vi "Teleop.vi"(10 "Match Info":T1={"Autonomous Elapsed Seconds"=0.0, "TeleOp Elapsed Seconds"=0.0, "Disabled Elapsed Seconds"=0.0, "Visited Autonomous"=FALSE, "Visited TeleOp"=FALSE, "Visited Disabled"=FALSE, "Autonomous Settings"={"Autonomous Style"=enum."Independent", "VI Refnum"=refnum}}, 11 "Call Context":T2) -> ()   [LabVIEW 2017]
doc: "This VI is called for each TeleOp packet received from the DS where the robot is not disabled. It is often used to read from the joysticks and update I/O or to update setpoints for timed control loops. It should complete and return within 20 milliseconds or it may miss DS packets."
uses:
  <vilib>/Rock Robotics/WPI/DriverStation/WPI_DriverStationDerivedRobotMode.ctl
  <vilib>/Rock Robotics/WPI/DriverStation/WPI_DriverStationMatch Info.ctl
  globals.vi
  <vilib>/Rock Robotics/WPI/Utilities/WPI_GetSetVariantRefNum.vi
  <vilib>/Rock Robotics/Network Tables/NT Write Boolean Array.vi
  <vilib>/Rock Robotics/Network Tables/NT Write Numeric Array.vi
  <vilib>/Rock Robotics/Network Tables/NT Read Boolean.vi
  <vilib>/Rock Robotics/Network Tables/NT Read Number.vi
panel:
  out "Sample Slider 0":dbl(slide) scale=0.0..5.0
  out "Sample Boolean 1":bool
  out "Sample Boolean 0":bool
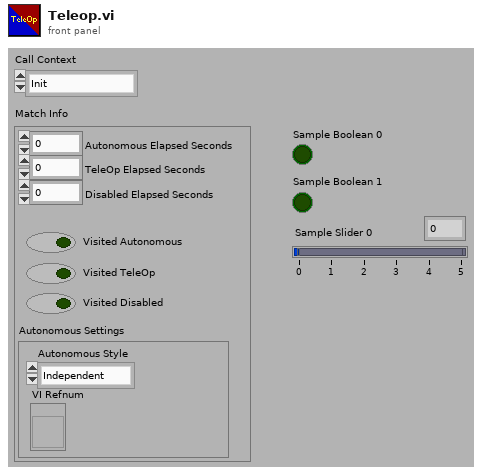
[diagram p1: front panel]
types:
  T1 = typedef "WPI_DriverStationMatch Info.ctl" = cluster{"Autonomous Elapsed Seconds":dbl, "TeleOp Elapsed Seconds":dbl, "Disabled Elapsed Seconds":dbl, "Visited Autonomous":bool, "Visited TeleOp":bool, "Visited Disabled":bool, "Autonomous Settings":cluster{"Autonomous Style":enum16{"Iterative", "Independent"}, "VI Refnum":refnum<vi>}}
  T2 = typedef "WPI_DriverStationDerivedRobotMode.ctl" = enum16{"Init", "Execute", "Stop"}
  T3 = typedef "WPI_JoystickDevRef.ctl" = cluster{"Device":T4}
  T4 = typedef "WPI_JoystickDeviceEnum.ctl" = enum16{"USB 0", "USB 1", "USB 2", "USB 3", "USB 4", "USB 5"}
  T5 = typedef "WPI_MotorControlDeviceRef.ctl" = cluster{"DeviceStatus":errorcluster, "Type":T6, "PWM":cluster{"PWM Channel":T7, "DeadBand":T8}, "CAN":cluster{"Device Number":u8, "SetOutput VI Ref":variant, "GetOutput VI Ref":variant, "Enable VI Ref":variant, "Disable VI Ref":variant, "Data":variant}, "Invert":bool, "DIO PWM":cluster{"PWM \"Enable\" Channel":T7, "DIOChannel":T9, "PWM Rate":dbl}}
  T6 = typedef "WPI_MotorControlType.ctl" = enum16{"PWM", "CAN", "DIO PWM"}
  T7 = typedef "FPGA_DIOPWMChannel.ctl" = enum8{"PWM 0", "PWM 1", "PWM 2", "PWM 3", "PWM 4", "PWM 5", "PWM 6", "PWM 7", "PWM 8", "PWM 9", "PWM MXP 0", "PWM MXP 1", "PWM MXP 2", "PWM MXP 3", "PWM MXP 4", "PWM MXP 5", "PWM MXP 6", "PWM MXP 7", "PWM MXP 8", "PWM MXP 9", "Invalid"}
  T8 = typedef "WPI_PWMDeadband.ctl" = cluster{"Name":string, "maxPositivePwm":i32, "minPositivePwm":i32, "centerPwm":i32, "maxNegativePwm":i32, "minNegativePwm":i32, "angularRange":u16}
  T9 = typedef "FPGA_DIOChannel.ctl" = enum8{"DIO 0", "DIO 1", "DIO 2", "DIO 3", "DIO 4", "DIO 5", "DIO 6", "DIO 7", "DIO 8", "DIO 9", "DIO MXP 0", "DIO MXP 1", "DIO MXP 2", "DIO MXP 3", "DIO MXP 4", "DIO MXP 5", "DIO MXP 6", "DIO MXP 7", "DIO MXP 8", "DIO MXP 9", "DIO MXP 10", "DIO MXP 11", "DIO MXP 12", "DIO MXP 13", "DIO MXP 14", "DIO MXP 15", "SPI Port CS1", "SPI Port CS2", "SPI Port CS3", "SPI Port MISO", "SPI Port MOSI", "Invalid"}
  T10 = cluster{"MotorControlDevRef":T5, "MotorControlDevRef":T5}
  T11 = typedef "WPI_AnalogChannelDevRef.ctl" = cluster{"DevStatus":errorcluster, "Analog Channel":T12}
  T12 = typedef "FPGA_AIChannel.ctl" = enum8{"AI 0", "AI 1", "AI 2", "AI 3", "AI MXP 0", "AI MXP 1", "AI MXP 2", "AI MXP 3", "Invalid"}
  T13 = typedef "WPI_EncoderDevRef.ctl" = cluster{"DevStatus":errorcluster, "EncoderIndex":T14, "CounterIndex":T15, "DistancePerCount":dbl, "Decoding Type":T16}
  T14 = typedef "FPGA_EncoderIdx.ctl" = enum8{"Enc 0", "Enc 1", "Enc 2", "Enc 3", "Enc 4", "Enc 5", "Enc 6", "Enc 7", "Invalid"}
  T15 = typedef "FPGA_CounterCtrSystemIndex.ctl" = enum8{"Ctr 0", "Ctr 1", "Ctr 2", "Ctr 3", "Ctr 4", "Ctr 5", "Ctr 6", "Ctr 7", "Invalid"}
  T16 = typedef "WPI_EncoderType.ctl" = enum16{"1x", "2x", "4x"}
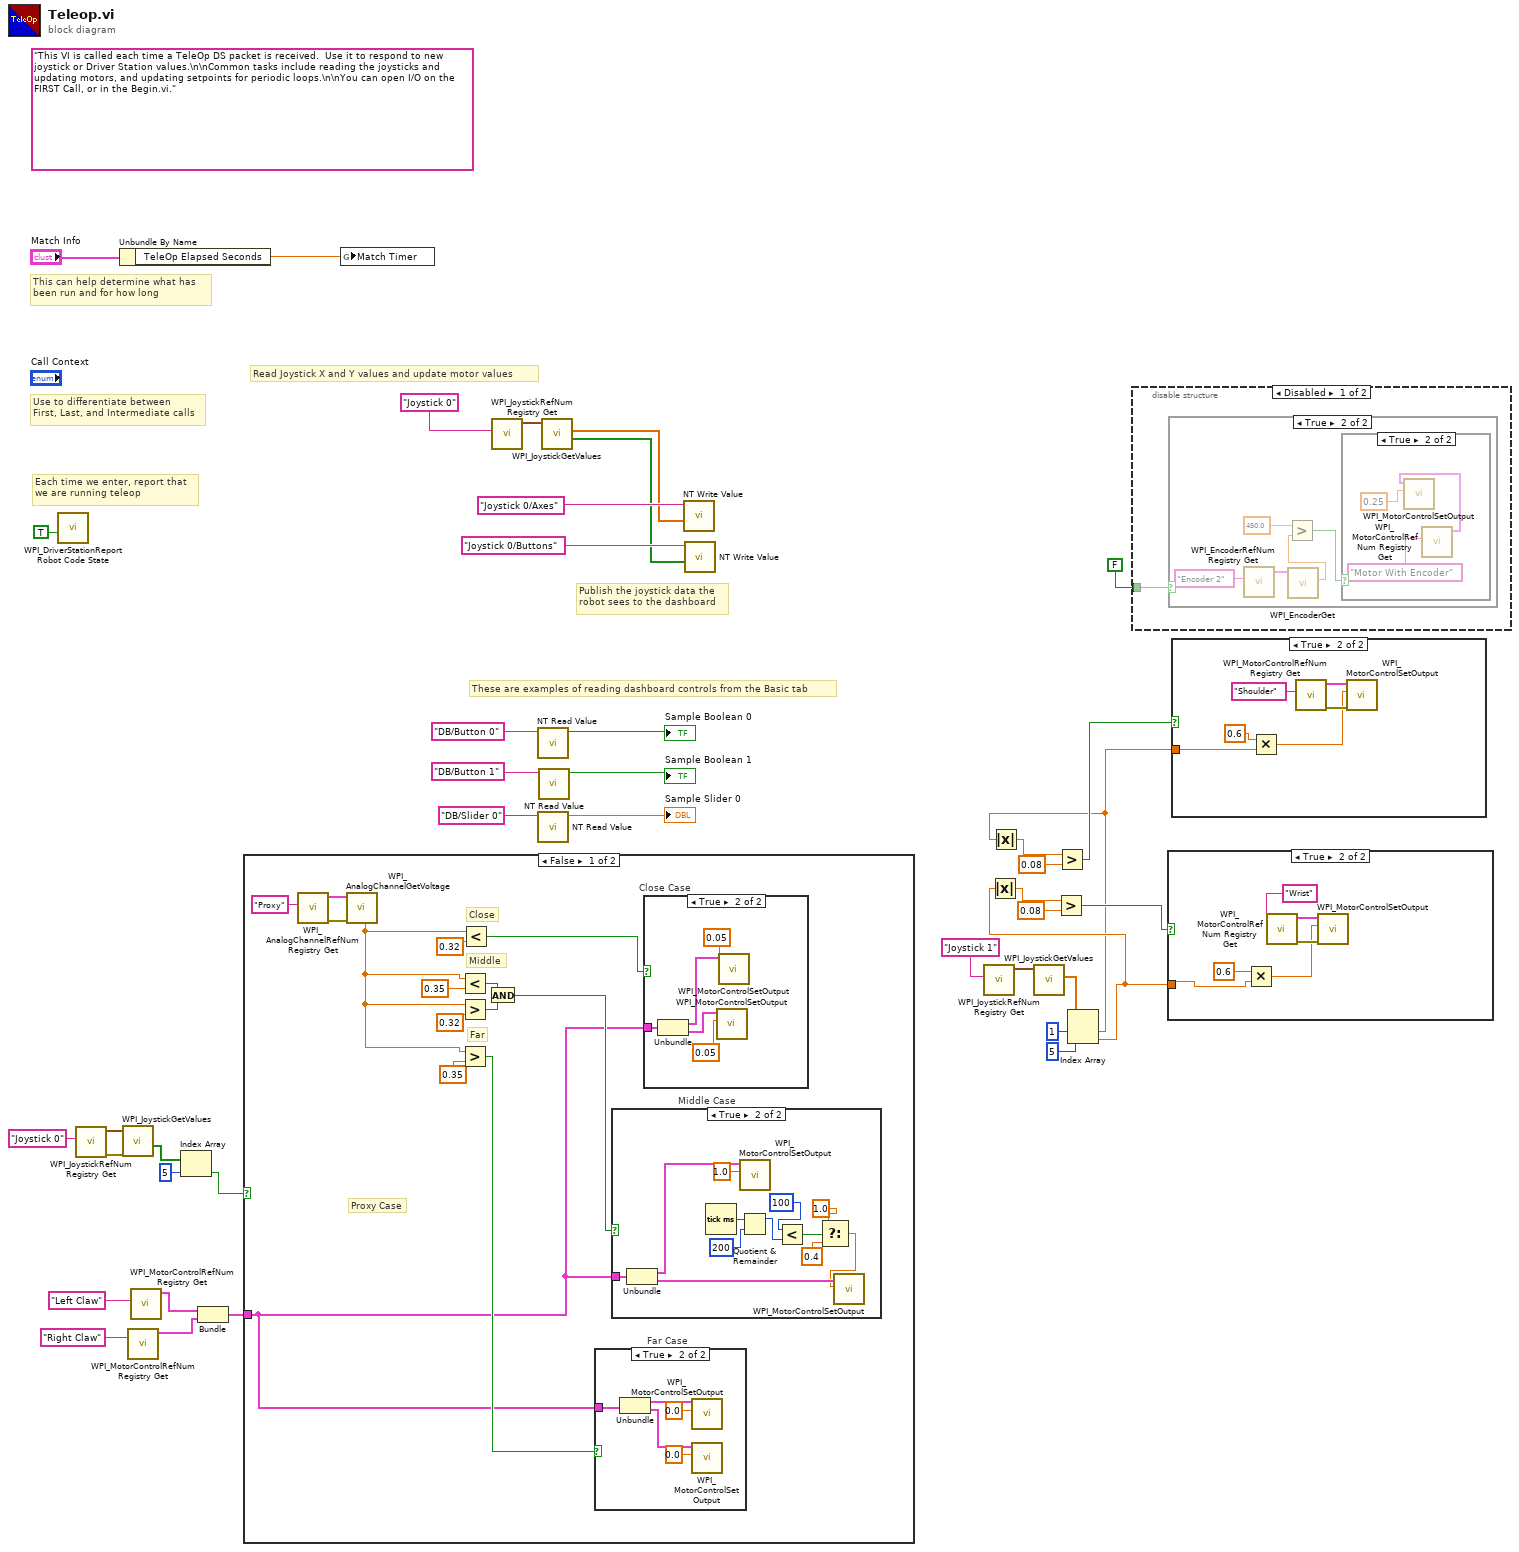
[diagram p0: block diagram]
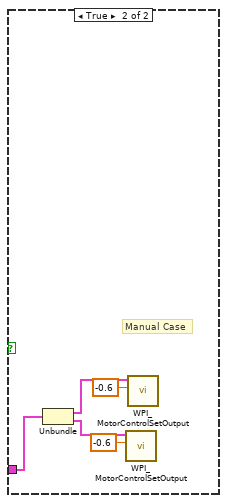
[diagram p5: hidden frame]
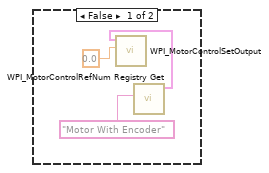
[diagram p7: hidden frame]
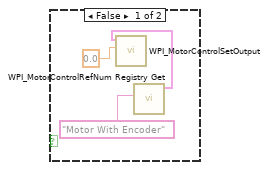
[diagram p8: hidden frame]
diagram:
  (unwired) "This VI is called each time a TeleOp DS packet is received.  Use it to respond to new joystick or Driver Station values.\n\nCommon tasks include reading the joysticks and updating motors, and updating setpoints for periodic loops.\n\nYou can open I/O on the FIRST Call, or in the Begin.vi."
  # "These are examples of reading dashboard controls from the Basic tab"
  # "Publish the joystick data the\nrobot sees to the dashboard"
  # "Each time we enter, report that\nwe are running teleop"
  # "Use to differentiate between\nFirst, Last, and Intermediate calls"
  # "This can help determine what has\nbeen run and for how long"
  # "Read Joystick X and Y values and update motor values"
  n1 = call <vilib>:"WPI_DriverStationReport Robot Code State.vi"("TeleOp"=TRUE ("Autonomous")) -> ()  [unwired: 10 in, 1 out]
  n2 = call <vilib>:"WPI_JoystickRefNum Registry Get.vi"("refnum name"="Joystick 0") -> ("error out"=w11:errorcluster, "JoystickDevRef"=w10:T3)  [unwired: 9 in]
  n3 = Unbundle By Name("Match Info") -> ("TeleOp Elapsed Seconds"=w25:dbl)
  n4 = call <vilib>:"WPI_JoystickGetValues.vi"("error in (no error)"=w11, "JoystickDevRef"=w10) -> ("Buttons"=w9:bool[])  [unwired: 5 in, 4 out]
  n5 = call <vilib>:"WPI_MotorControlRefNum Registry Get.vi"("refnum name"="Right Claw") -> ("MotorControlDevRef"=w4:T5)  [unwired: 9 in, 1 out]
  n6 = call <vilib>:"WPI_MotorControlRefNum Registry Get.vi"("refnum name"="Left Claw") -> ("MotorControlDevRef"=w3:T5)  [unwired: 9 in, 1 out]
  n7 = Index Array(array=w9, index=5) -> (element=w7:bool)
  n8 = Bundle("MotorControlDevRef"=w3, "MotorControlDevRef"=w4) -> (w2:T10)  [unwired: 1 in]
  n9 = case shown="False" w7 {
    tunnel: w2 -> [w41 w79]
    frame False {
      # "Proxy Case"
      # "Close"
      # "Middle"
      # "Far"
      n10 = call <vilib>:"WPI_AnalogChannelRefNum Registry Get.vi"("refnum name"="Proxy") -> ("error out"=w53:errorcluster, "AIDeviceRef"=w52:T11)  [unwired: 9 in]
      n11 = call <vilib>:"WPI_AnalogChannelGetVoltage.vi"("error in (no error)"=w53, "AIDeviceRef"=w52) -> ("Voltage"=w46:dbl)  [unwired: 7 in, 2 out]
      n12 = Less?(x=w46, y=0.35) -> (x < y?=w51:bool)
      n13 = Greater?(x=w46, y=0.32) -> (0:w50:bool)
      n14 = Greater?(x=w46, y=0.35) -> (0:w45:bool)
      n15 = Less?(x=w46, y=0.32) -> (x < y?=w43:bool)
      n16 = And(x=w51, y=w50) -> (x .and. y?=w44:bool)
      n17 = case "Far Case" shown="True" w45 {
        tunnel: w41 -> [_ w59]
        frame False {
        }
        frame True {
          n18 = Unbundle(w59) -> ("MotorControlDevRef"=w58:T5, "MotorControlDevRef"=w57:T5)
          n19 = call <vilib>:"WPI_MotorControlSetOutput.vi"("Output"=0.0, "MotorControlDevRef"=w58) -> ()  [unwired: 7 in, 3 out]
          n20 = call <vilib>:"WPI_MotorControlSetOutput.vi"("Output"=0.0, "MotorControlDevRef"=w57) -> ()  [unwired: 7 in, 3 out]
        }
      }
      n21 = case "Middle Case" shown="True" w44 {
        tunnel: w41 -> [_ w71]
        frame False {
        }
        frame True {
          n22 = Unbundle(w71) -> ("MotorControlDevRef"=w70:T5, "MotorControlDevRef"=w69:T5)
          n23 = Tick Count (ms)() -> (millisecond timer value=w65:u32)
          n24 = call <vilib>:"WPI_MotorControlSetOutput.vi"("Output"=1.0, "MotorControlDevRef"=w70) -> ()  [unwired: 7 in, 3 out]
          n25 = Quotient & Remainder(x=w65, y=u32 200) -> (x-y*floor(x/y)=w66:u32)  [unwired: 1 out]
          n26 = Less?(x=u32 100, y=w66) -> (x < y?=w67:bool)
          n27 = Select(t=1.0, s=w67, f=0.4) -> (s? t:f=w60:dbl)
          n28 = call <vilib>:"WPI_MotorControlSetOutput.vi"("Output"=w60, "MotorControlDevRef"=w69) -> ()  [unwired: 7 in, 3 out]
        }
      }
      n29 = case "Close Case" shown="True" w43 {
        tunnel: w41 -> [_ w76]
        frame False {
        }
        frame True {
          n30 = Unbundle(w76) -> ("MotorControlDevRef"=w75:T5, "MotorControlDevRef"=w74:T5)
          n31 = call <vilib>:"WPI_MotorControlSetOutput.vi"("Output"=0.05, "MotorControlDevRef"=w74) -> ()  [unwired: 7 in, 3 out]
          n32 = call <vilib>:"WPI_MotorControlSetOutput.vi"("Output"=0.05, "MotorControlDevRef"=w75) -> ()  [unwired: 7 in, 3 out]
        }
      }
    }
    frame True {
      # "Manual Case"
      n33 = Unbundle(w79) -> ("MotorControlDevRef"=w81:T5, "MotorControlDevRef"=w80:T5)
      n34 = call <vilib>:"WPI_MotorControlSetOutput.vi"("Output"=-0.6, "MotorControlDevRef"=w80) -> ()  [unwired: 7 in, 3 out]
      n35 = call <vilib>:"WPI_MotorControlSetOutput.vi"("Output"=-0.6, "MotorControlDevRef"=w81) -> ()  [unwired: 7 in, 3 out]
    }
  }
  n36 = global write "globals.vi" "Match Timer"(w25) -> ()
  n37 = call <vilib>:"WPI_JoystickRefNum Registry Get.vi"("refnum name"="Joystick 0") -> ("JoystickDevRef"=w38:T3)  [unwired: 1 in, 9 out]
  n38 = call-poly <vilib>:"NT Read Value.vi"("Name"="DB/Button 0" ("refnum name")) -> ("Boolean"=→"Sample Boolean 0":bool)  [unwired: 9 in, 1 out]
  n39 = call-poly <vilib>:"NT Read Value.vi"("Name"="DB/Slider 0" ("refnum name")) -> ("Numeric"=→"Sample Slider 0":dbl)  [unwired: 9 in, 1 out]
  n40 = call-poly <vilib>:"NT Read Value.vi"("Name"="DB/Button 1" ("refnum name")) -> ("Boolean"=→"Sample Boolean 1":bool)  [unwired: 9 in, 1 out]
  n41 = call <vilib>:"WPI_JoystickGetValues.vi"("JoystickDevRef"=w38) -> ("Buttons"=w33:bool[], "Axes"=w34:dbl[])  [unwired: 6 in, 3 out]
  n42 = call-poly <vilib>:"NT Write Value.vi"("Numeric Array"=w34, "Name"="Joystick 0/Axes") -> ()  [unwired: 9 in, 1 out]
  n43 = call-poly <vilib>:"NT Write Value.vi"("Boolean Array"=w33, "Name"="Joystick 0/Buttons") -> ()  [unwired: 9 in, 1 out]
  n44 = call <vilib>:"WPI_JoystickRefNum Registry Get.vi"("refnum name"="Joystick 1") -> ("JoystickDevRef"=w24:T3)  [unwired: 1 in, 9 out]
  n45 = call <vilib>:"WPI_JoystickGetValues.vi"("JoystickDevRef"=w24) -> ("Axes"=w20:dbl[])  [unwired: 6 in, 4 out]
  n46 = Index Array(array=w20, index #1=1 ("index"), index #2=5 ("index")) -> (element #1=w1:dbl, element #2=w16:dbl)
  n47 = Absolute Value(x=w16) -> (abs(x)=w15:dbl)
  n48 = Absolute Value(x=w1) -> (abs(x)=w19:dbl)
  n49 = Greater?(x=w15, y=0.08) -> (0:w13:bool)
  n50 = Greater?(x=w19, y=0.08) -> (0:w17:bool)
  n51 = disable-structure shown="Disabled" {
    disable-tunnel: FALSE -> [w82 _]
    frame Disabled {
      n52 = case shown="True" w82 {
        frame False {
          n53 = call <vilib>:"WPI_MotorControlRefNum Registry Get.vi"("refnum name"="Motor With Encoder") -> ("MotorControlDevRef"=w83:T5)  [unwired: 9 in, 1 out]
          n54 = call <vilib>:"WPI_MotorControlSetOutput.vi"("Output"=0.0, "MotorControlDevRef"=w83) -> ()  [unwired: 7 in, 3 out]
        }
        frame True {
          n55 = call <vilib>:"WPI_EncoderRefNum Registry Get.vi"("refnum name"="Encoder 2") -> ("EncoderDevRef"=w89:T13)  [unwired: 9 in, 1 out]
          n56 = call <vilib>:"WPI_EncoderGet.vi"("EncoderDevRef"=w89) -> ("Distance"=w86:dbl)  [unwired: 5 in, 5 out]
          n57 = Greater?(x=450.0, y=w86) -> (0:w88:bool)
          n58 = case shown="True" w88 {
            frame False {
              n59 = call <vilib>:"WPI_MotorControlRefNum Registry Get.vi"("refnum name"="Motor With Encoder") -> ("MotorControlDevRef"=w91:T5)  [unwired: 9 in, 1 out]
              n60 = call <vilib>:"WPI_MotorControlSetOutput.vi"("Output"=0.0, "MotorControlDevRef"=w91) -> ()  [unwired: 7 in, 3 out]
            }
            frame True {
              n61 = call <vilib>:"WPI_MotorControlRefNum Registry Get.vi"("refnum name"="Motor With Encoder") -> ("MotorControlDevRef"=w94:T5)  [unwired: 9 in, 1 out]
              n62 = call <vilib>:"WPI_MotorControlSetOutput.vi"("Output"=0.25, "MotorControlDevRef"=w94) -> ()  [unwired: 7 in, 3 out]
            }
          }
        }
      }
    }
    frame Enabled {
    }
  }
  n63 = case shown="True" w13 {
    tunnel: w16 -> [_ w97]
    frame False {
    }
    frame True {
      n64 = Multiply(x=0.6, y=w97) -> (x*y=w100:dbl)
      n65 = call <vilib>:"WPI_MotorControlRefNum Registry Get.vi"("refnum name"="Wrist") -> ("error out"=w102:errorcluster, "MotorControlDevRef"=w101:T5)  [unwired: 9 in]
      n66 = call <vilib>:"WPI_MotorControlSetOutput.vi"("error in (no error)"=w102, "Output"=w100, "MotorControlDevRef"=w101) -> ()  [unwired: 6 in, 3 out]
    }
  }
  n67 = case shown="True" w17 {
    tunnel: w1 -> [_ w103]
    frame False {
    }
    frame True {
      n68 = Multiply(x=0.6, y=w103) -> (x*y=w104:dbl)
      n69 = call <vilib>:"WPI_MotorControlRefNum Registry Get.vi"("refnum name"="Shoulder") -> ("error out"=w107:errorcluster, "MotorControlDevRef"=w106:T5)  [unwired: 9 in]
      n70 = call <vilib>:"WPI_MotorControlSetOutput.vi"("error in (no error)"=w107, "Output"=w104, "MotorControlDevRef"=w106) -> ()  [unwired: 6 in, 3 out]
    }
  }
